vi "zero flow sensor.vi"(3 "Sensor index":u32, 4 "data memory (s)":sgl format="%.3f") -> ()   [LabVIEW 2010]
uses:
  DAQ configuration/Sensor buffer command.ctl
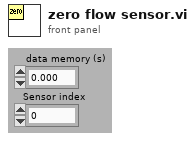
[diagram p1: front panel]
types:
  T1 = typedef "Sensor buffer command.ctl" = enum16{"read average", "read recent", "read all", "write", "configure", "clear"}
  T2 = typedef "Sensor data.ctl" = cluster{" Sensor array":T3[], "Time":dbl}
  T3 = typedef "sensor cluster.ctl" = cluster{"voltage":sgl, "scaled":sgl, "units":string, "Out of Range":bool}
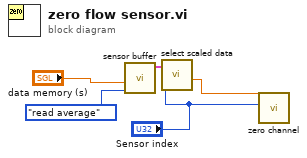
[diagram p0: block diagram]
diagram:
  n1 = call "sensor buffer.vi"("command"=Sensor_buffer_command."read average", "smooth interval (s)"="data memory (s)") -> ("Sensor Data smoothed"=w4:T2)  [unwired: 3 in, 2 out]
  n2 = call "select scaled data.vi"("Sensor index"="Sensor index", "Sensor Data"=w4) -> ("voltage"=w5:sgl)  [unwired: 4 in, 5 out]
  n3 = call "zero channel.vi"("Index"="Sensor index", "Mean (Volts)"=w5) -> ()  [unwired: 6 in]
